vi "Index.vi"(10 "Shoot":bool, 11 "Outputdisabled":dbl=-0.007874015748031496 format="%#_13g") -> ()   [LabVIEW 2016]
panel:
  in  "Output":dbl=-0.007874015748031496 format="%#_13g"
  in  "Shoot 2":bool
  in  "Max Effort":dbl=0.5 format="%#_13g"
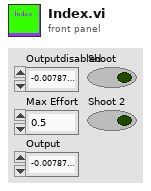
[diagram p1: front panel]
types:
  T1 = typedef "WPI_MotorControlDeviceRef.ctl" = cluster{"DeviceStatus":errorcluster, "Type":T2, "PWM":cluster{"PWM Channel":T3, "DeadBand":T4}, "CAN":cluster{"Device Number":u8, "SetOutput VI Ref":variant, "GetOutput VI Ref":variant, "Enable VI Ref":variant, "Disable VI Ref":variant, "Data":variant}, "Invert":bool}
  T2 = typedef "WPI_MotorControlType.ctl" = enum16{"PWM", "CAN"}
  T3 = typedef "FPGA_DIOPWMChannel.ctl" = enum8{"PWM 0", "PWM 1", "PWM 2", "PWM 3", "PWM 4", "PWM 5", "PWM 6", "PWM 7", "PWM 8", "PWM 9", "PWM MXP 0", "PWM MXP 1", "PWM MXP 2", "PWM MXP 3", "PWM MXP 4", "PWM MXP 5", "PWM MXP 6", "PWM MXP 7", "PWM MXP 8", "PWM MXP 9", "Invalid"}
  T4 = typedef "WPI_PWMDeadband.ctl" = cluster{"Name":string, "maxPositivePwm":i32, "minPositivePwm":i32, "centerPwm":i32, "maxNegativePwm":i32, "minNegativePwm":i32, "angularRange":u16}
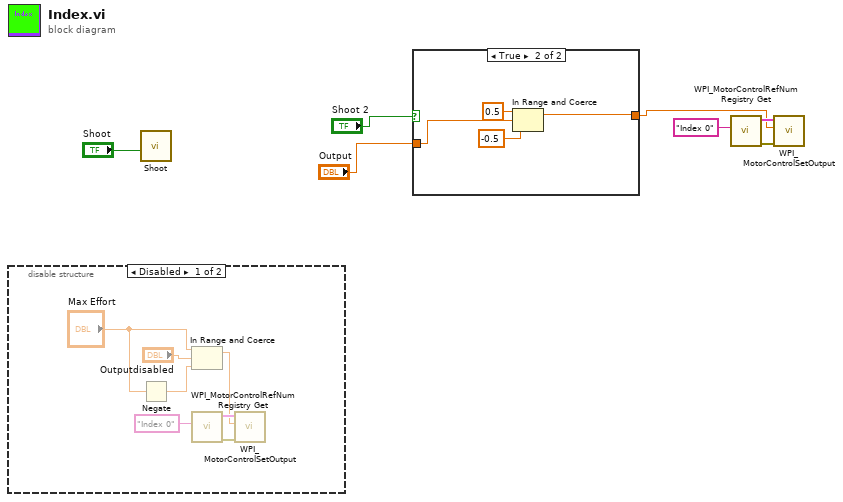
[diagram p0: block diagram]
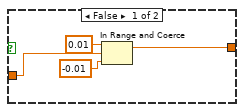
[diagram p2: hidden frame]
diagram:
  n1 = disable-structure shown="Disabled" {
    frame Disabled {
      n2 = Negate(x="Max Effort") -> (-x=w9:dbl)
      n3 = In Range and Coerce(upper limit="Max Effort", x="Outputdisabled", lower limit=w9) -> (coerced(x)=w10:dbl)  [unwired: 1 out]
      n4 = call <vilib>:"WPI_MotorControlRefNum Registry Get.vi"("refnum name"="Index 0") -> ("error out"=w13:errorcluster, "MotorControlDevRef"=w14:T1)  [unwired: 9 in]
      n5 = call <vilib>:"WPI_MotorControlSetOutput.vi"("error in (no error)"=w13, "Output"=w10, "MotorControlDevRef"=w14) -> ()  [unwired: 6 in, 3 out]
    }
    frame Enabled {
    }
  }
  n6 = call "Shoot.vi"("Shoot"="Shoot") -> ()  [unwired: 10 in]
  n7 = case shown="True" "Shoot 2" {
    tunnel: "Output" -> [w18 w22]
    tunnel: [w15 w19] -> w1
    frame False {
      n8 = In Range and Coerce(upper limit=0.01, x=w18, lower limit=-0.01 ("upper limit")) -> (coerced(x)=w15:dbl)  [unwired: 1 out]
    }
    frame True {
      n9 = In Range and Coerce(upper limit=0.5, x=w22, lower limit=-0.5 ("upper limit")) -> (coerced(x)=w19:dbl)  [unwired: 1 out]
    }
  }
  n10 = call <vilib>:"WPI_MotorControlRefNum Registry Get.vi"("refnum name"="Index 0") -> ("error out"=w3:errorcluster, "MotorControlDevRef"=w2:T1)  [unwired: 9 in]
  n11 = call <vilib>:"WPI_MotorControlSetOutput.vi"("error in (no error)"=w3, "Output"=w1, "MotorControlDevRef"=w2) -> ()  [unwired: 6 in, 3 out]
